vi "Rapid Read_NI_Done.vi"(0 "NI Card":refnum<k15> caption="instrument handle", 1 "Motion Settings In":T1={"No Motion?"=FALSE, "Motion System"=enum."NI 735x", "Motion Bd ID"=1, "Motion Profile"="SMAC1", "# Axis"=1, "Reverse Z axis?"=TRUE, "SMAC Axis"=0, "scan pair"=enum."y-(x) scan", "RT fps"=6.0, "Steps per mm"=[1000, 1000, 1000, 1000], "Motor Parameters"={"velocity ct/s"=[10000.0, 10000.0, 10000.0, 50000.0], "accel ct/s^2"=[50000.0, 50000.0, 50000.0, 200000.0]}, "One Way Scan"=FALSE, "Reverse One Way Scan"=FALSE, "Global Position (mm)"=[], "Plane"=0, "Distance between\nscan lines (um)"=0.0, "Distance between\nscan planes (um)"=0.0, "number of scan planes"=1, "Total steps in line"=0, "Xtra plane\ndistance  (um)"=100, "Xtra planes "=1, "Add Axis"=FALSE, "overshoot cts"=200, "BKPT Shift"=0, "Scan Start Time (ms)"=0, "ESP VISA"="GPIB::1::INSTR", "3rd Axis"=1, "GL Ref Out"=refnum, "Galil Address"=""} {"3rd Axis" items=["x", "y", "z", "w"]; "Xtra planes" min=1; "Xtra plane\ndistance  (um)" min=0; "Distance between\nscan planes (um)" format="%.2f"; "Distance between\nscan lines (um)" format="%.2f"; "SMAC Axis" items=["None"=0, "Axis 1"=1, "Axis 2"=2, "Axis 3"=3, "Axis 4"=4, "Axis 5"=5, "Axis 6"=6, "Axis 7"=7, "Axis 8"=8, "Vector Space 1"=17, "Vector Space 2"=18, "Vector Space 3"=19, "Vector Space 4"=20]; "Motion Bd ID" min=1 max=32 step=1}, 9 "records":i32, 11 "error in":errorcluster, 14 "Pause?":bool) -> (6 "Reverse?":bool, 15 "error out":errorcluster)   [LabVIEW 2022 SP3]
uses:
  Motion Controllers/NI_controller/-NI_MotionRoutines/MotionParameters.ctl
  Motion Controllers/NI_controller/-NI_MotionRoutines/MotionSys.ctl
  Motion Controllers/-MotionRoutines/ScanAxis.ctl
  Motion Controllers/-MotionRoutines/3rdAxis.ctl
  Motion Controllers/Galil/Command Menu.ctl
  <vilib>/DAQmx/write.llb/DAQmx Write (Digital Bool 1Line 1Point).vi
  Motion Controllers/-MotionRoutines/MotionGlobals.vi
  <vilib>/DAQmx/miscellaneous.llb/DAQmx Fill In Error Info.vi
panel:
  # "1-D and 2-D B scan settings"
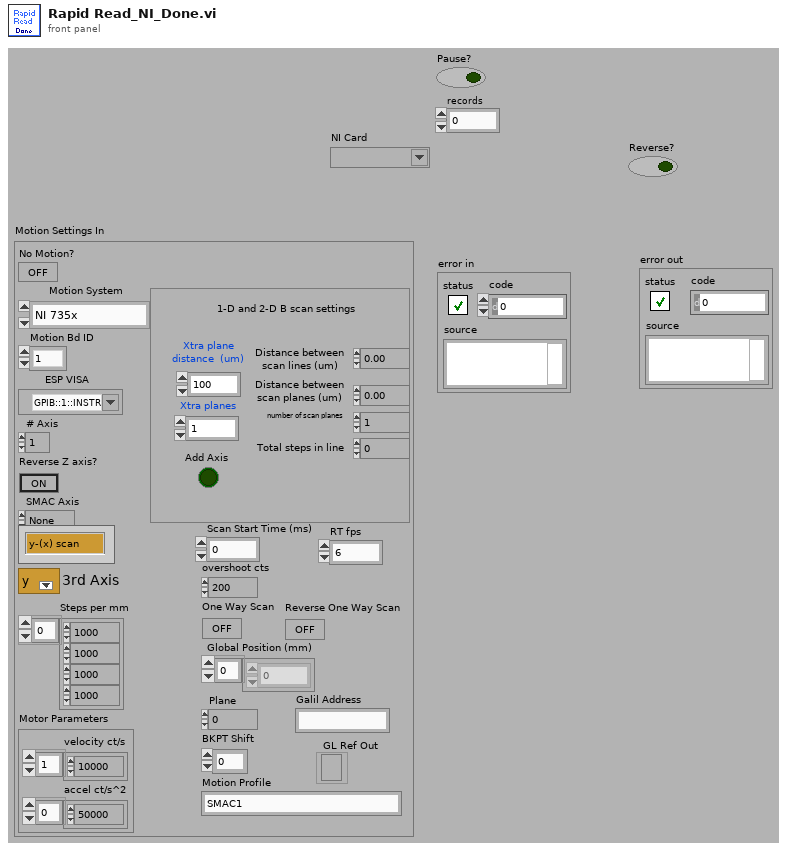
[diagram p1: front panel]
types:
  T1 = typedef "MotionParameters.ctl" = cluster{"No Motion?":bool, "Motion System":T2, "Motion Bd ID":u8, "Motion Profile":string, "# Axis":i8, "Reverse Z axis?":bool, "SMAC Axis":u16, "scan pair":T3, "RT fps":sgl, "Steps per mm":i32[], "Motor Parameters":cluster{"velocity ct/s":dbl[], "accel ct/s^2":dbl[]}, "One Way Scan":bool, "Reverse One Way Scan":bool, "Global Position (mm)":dbl[], "Plane":i32, "Distance between\nscan lines (um)":sgl, "Distance between\nscan planes (um)":sgl, "number of scan planes":i32, "Total steps in line":i32, "Xtra plane\ndistance  (um)":i32, "Xtra planes ":i32, "Add Axis":bool, "overshoot cts":i32, "BKPT Shift":i32, "Scan Start Time (ms)":u32, "ESP VISA":refnum<visa-resource-name>, "3rd Axis":T4, "GL Ref Out":refnum<k7>, "Galil Address":string}
  T2 = typedef "MotionSys.ctl" = enum16{"MM3000", "NI 735x", "Newport ESP", "No Motion Card", "Galil"}
  T3 = typedef "ScanAxis.ctl" = enum16{"y-(x) scan", "x-(y) scan", "z-(x) scan", "z-(y) scan", "y-(z) scan", "x-(z) scan", "w-(x) scan", "w-(y) scan", "w-(z) scan", "x-(w) scan", "y-(w) scan", "z-(w) scan"}
  T4 = typedef "3rdAxis.ctl" = u16
  T5 = typedef "Command Menu.ctl" = enum16{"CommandPassThrough", "Abort Motion", "Define Pos", "Velocity", "Acceleration", "Deceleration", "Position Rel", "Postion Abs", "Begin Move", "After Move", "Home", "KI", "KD", "KP", "IL", "Config I/O", "Set Bit", "Clear Bit", "Motor Off", "Moto On", "Status", "Execute", "Halt Execute", "HX Status", "Tell Velocity", "Check Motion", "BreakPoint", "Tell Position", "Current Code Line", "Tell Switches", "OC Force On", "OC Off", "Pos Soft Limit", "Rev Soft Limit"}
  T6 = typedef "Var" = u8
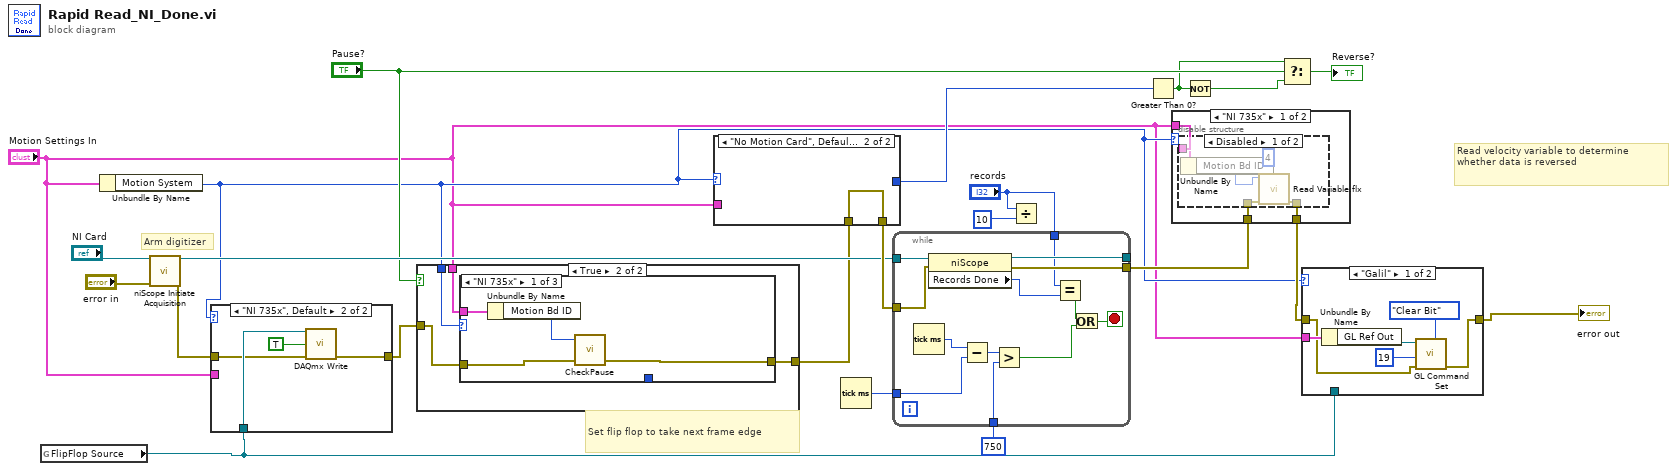
[diagram p0: block diagram]
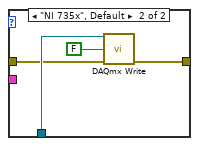
[diagram p2: hidden frame]
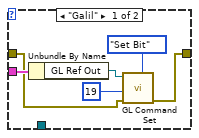
[diagram p3: hidden frame]
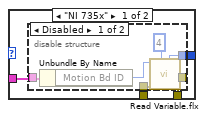
[diagram p6: hidden frame]
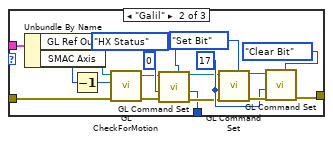
[diagram p9: hidden frame]
diagram:
  # "Arm digitizer"
  # "Set flip flop to take next frame edge"
  # "Read velocity variable to determine whether data is reversed"
  n1 = global read "MotionGlobals.vi" "FlipFlop Source"() -> (w4:refnum<k21>)
  n2 = Unbundle By Name("Motion Settings In") -> ("Motion System"=w2:T2)
  n3 = call <instrlib>:"niScope Initiate Acquisition.vi"("instrument handle"="NI Card", "error in"="error in") -> ("instrument handle out"=w15:refnum<k15>, "error out"=w6:errorcluster)  [unwired: 1 in, 11 out]
  n4 = case shown="\"NI 735x\", Default" w2 {
    tunnel: [w26 w31] -> w7
    tunnel: w4 -> [_ w30]
    tunnel: w6 -> [w23 w29]
    tunnel: "Motion Settings In" -> [w25 _]
    frame "Galil" {
      n5 = Unbundle By Name(w25) -> ("GL Ref Out"=w24:refnum<k7>)
      n6 = call "GL Command Set.vi"("Command"=Command_Menu."Set Bit", "error in (no error)"=w23, "Value"=19, "Galil.IGalil"=w24) -> ("error out"=w26:errorcluster)  [unwired: 3 in, 4 out]
    }
    frame "NI 735x", Default {
      n7 = call-poly <vilib>:"DAQmx Write.vi"("task/channels in"=w30, "data"=TRUE ("stop (T)"), "error in"=w29) -> ("error out"=w31:errorcluster)  [unwired: 10 in, 2 out]
    }
  }
  n8 = case shown="True" "Pause?" {
    tunnel: w7 -> [w33 w37]
    tunnel: [w33 w34] -> w14
    tunnel: w2 -> [_ w36]
    tunnel: "Motion Settings In" -> [_ w35]
    frame False {
    }
    frame True {
      n9 = case shown="\"NI 735x\"" w36 {
        tunnel: [w41 w55 w60] -> w34
        tunnel: w37 -> [w40 w58 w60]
        tunnel: w35 -> [w39 w51 _]
        tunnel: [_ w42 _] -> _
        frame "NI 735x" {
          n10 = Unbundle By Name(w39) -> ("Motion Bd ID"=w38:u8)
          n11 = call "CheckPause.vi"("error in"=w40, "Motion Board ID"=w38) -> ("error out"=w41:errorcluster)  [unwired: 3 in]
        }
        frame "Galil" {
          w52 = 17 ("Value")
          n12 = Unbundle By Name(w51) -> ("GL Ref Out"=w50:refnum<k7>, "SMAC Axis"=w49:u16)
          n13 = Decrement(x=w49) -> (x-1=w59:u16)
          n14 = call "GL CheckForMotion.vi"("error in"=w58, "Axis"=w59, "Refnum in"=w50) -> ("error out"=w46:errorcluster, "Refnum out"=w43:refnum<k7>)  [unwired: 6 in, 1 out]
          n15 = call "GL Command Set.vi"("Command"=Command_Menu."HX Status", "error in (no error)"=w46, "Value"=0, "Galil.IGalil"=w43) -> ("error out"=w45:errorcluster, "Response#"=w42:i32, "ref out"=w44:refnum<k7>)  [unwired: 3 in, 2 out]
          n16 = call "GL Command Set.vi"("Command"=Command_Menu."Set Bit", "error in (no error)"=w45, "Value"=w52, "Galil.IGalil"=w44) -> ("error out"=w56:errorcluster, "ref out"=w53:refnum<k7>)  [unwired: 3 in, 3 out]
          n17 = call "GL Command Set.vi"("Command"=Command_Menu."Clear Bit", "error in (no error)"=w56, "Value"=w52, "Galil.IGalil"=w53) -> ("error out"=w55:errorcluster)  [unwired: 3 in, 4 out]
        }
        frame "No Motion Card", Default {
        }
      }
    }
  }
  n18 = case shown="\"No Motion Card\", Default" w2 {
    tunnel: [w64 w71] -> w17
    tunnel: [w63 _] -> w16
    tunnel: w14 -> [w62 w71]
    tunnel: "Motion Settings In" -> [w61 _]
    frame "NI 735x" {
      n19 = disable-structure shown="Disabled" {
        disable-tunnel: [w69 _] -> w64
        disable-tunnel: [w68 _] -> w63
        disable-tunnel: w62 -> [w67 _]
        disable-tunnel: w61 -> [w66 _]
        frame Disabled {
          n20 = Unbundle By Name(w66) -> ("Motion Bd ID"=w65:u8)
          n21 = call <vilib>:"Read Variable.flx"("Var"=T6 4, "error in (no error)"=w67, "Board ID"=w65) -> ("error out"=w69:errorcluster, "Output"=w68:i32)  [unwired: 1 in, 4 out]
        }
        frame Enabled {
        }
      }
    }
    frame "No Motion Card", Default {
    }
  }
  n22 = Tick Count (ms)() -> (millisecond timer value=w20:u32)
  n23 = while {
    tunnel: w15 -> [w84]
    tunnel: [w83] -> _
    tunnel: w17 -> [w82]
    tunnel: [w81] -> w18
    tunnel: w20 -> [w79]
    tunnel: u32 750 ("y") -> [w77]
    tunnel: "records" -> [w72]
    stop <- w75 stop-if-true
    n24 = Tick Count (ms)() -> (millisecond timer value=w80:u32)
    n25 = property class="niScope"(reference=w84, error in=w82) -> (reference out=w83:refnum<k15>, error out=w81:errorcluster, "Records Done"=w74:i32)
    n26 = Subtract(x=w80, y=w79) -> (x-y=w78:u32)
    n27 = Greater?(x=w78, y=w77) -> (0:w76:bool)
    n28 = Equal?(x=w72, y=w74) -> (x = y?=w73:bool)
    n29 = Or(x=w73, y=w76) -> (x .or. y?=w75:bool)
  }
  n30 = Divide(x="records", y=10 ("x")) -> ()  [unwired: 1 out]
  n31 = Greater Than 0?(x=w16) -> (x > 0?=w12:bool)
  n32 = case shown="\"NI 735x\"" w2 {
    tunnel: w18 -> [w87 w93]
    tunnel: [w86 w93] -> w3
    tunnel: "Motion Settings In" -> [w85 _]
    frame "NI 735x" {
      n33 = disable-structure shown="Disabled" {
        disable-tunnel: w87 -> [w91 _]
        disable-tunnel: [w90 _] -> w86
        disable-tunnel: w85 -> [w89 _]
        frame Disabled {
          n34 = Unbundle By Name(w89) -> ("Motion Bd ID"=w88:u8)
          n35 = call <vilib>:"Read Variable.flx"("Var"=T6 4, "error in (no error)"=w91, "Board ID"=w88) -> ("error out"=w90:errorcluster)  [unwired: 1 in, 5 out]
        }
        frame Enabled {
        }
      }
    }
    frame "No Motion Card", Default {
    }
  }
  n36 = Not(x=w12) -> (.not. x?=w11:bool)
  n37 = Select(t=w12, s="Pause?", f=w11) -> (s? t:f=→"Reverse?":bool)
  n38 = case shown="\"Galil\"" w2 {
    tunnel: [w95 w102] -> w5
    tunnel: w4 -> [_ w101]
    tunnel: w3 -> [w94 w100]
    tunnel: "Motion Settings In" -> [w96 _]
    frame "Galil" {
      n39 = Unbundle By Name(w96) -> ("GL Ref Out"=w99:refnum<k7>)
      n40 = call "GL Command Set.vi"("Command"=Command_Menu."Clear Bit", "error in (no error)"=w94, "Value"=19, "Galil.IGalil"=w99) -> ("error out"=w95:errorcluster)  [unwired: 3 in, 4 out]
    }
    frame "NI 735x", Default {
      n41 = call-poly <vilib>:"DAQmx Write.vi"("task/channels in"=w101, "data"=FALSE ("stop (T)"), "error in"=w100) -> ("error out"=w102:errorcluster)  [unwired: 10 in, 2 out]
    }
  }
  "error out" <- w5
